vi "Auto Trans.vi"(0 "Scene Object In":refnum<vi>, 1 "Psi":dbl(slide) step=1.0 scale=-110.0..110.0, 2 "Psi i":dbl(slide) step=1.0 scale=-110.0..110.0, 3 "Boolean":bool, 5 "Base":refnum<vi>, 7 "Gimbal":refnum<vi>, 9 "Telescope":refnum<vi>, 11 "error in (no error)":errorcluster, 12 "Theta":dbl(slide) step=1.0 scale=-110.0..110.0, 13 "Theta i":dbl(slide) step=1.0 scale=-110.0..110.0) -> (4 "Scene Object Out":refnum<vi>, 15 "error out":errorcluster)   [LabVIEW 2015]
uses:
  <vilib>/picture/3D Picture Control/NI_3D Picture Control.lvlib
panel:
  out "Delta Psi 2":dbl
  out "Delta Psi":dbl
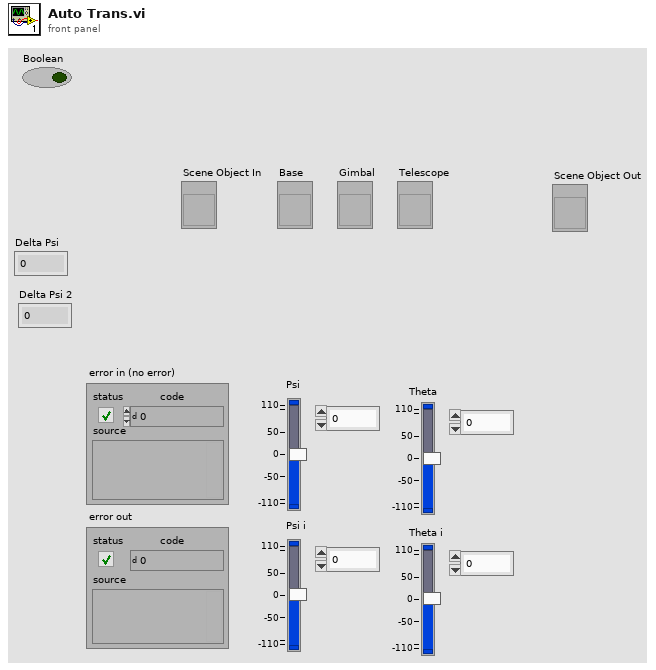
[diagram p1: front panel]
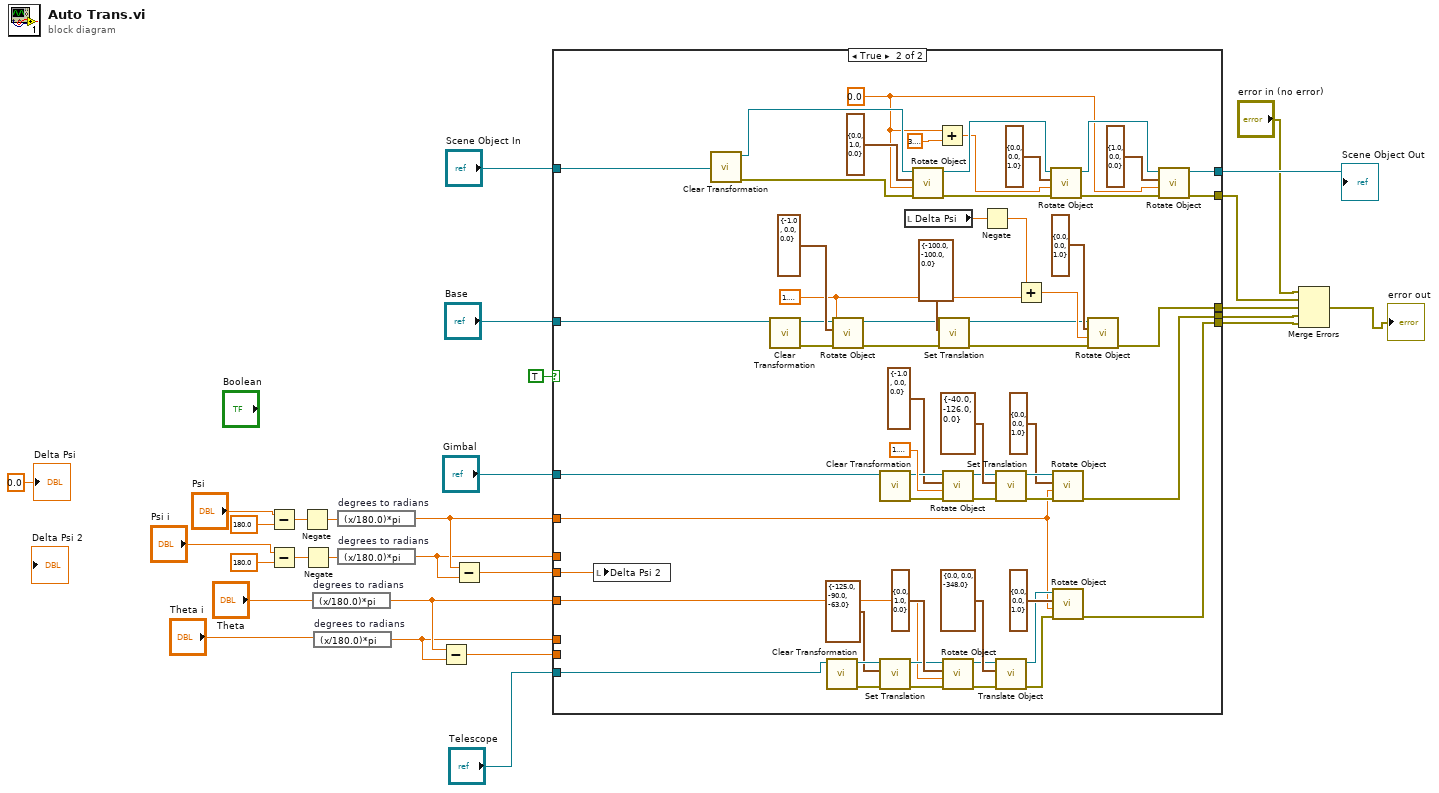
[diagram p0: block diagram]
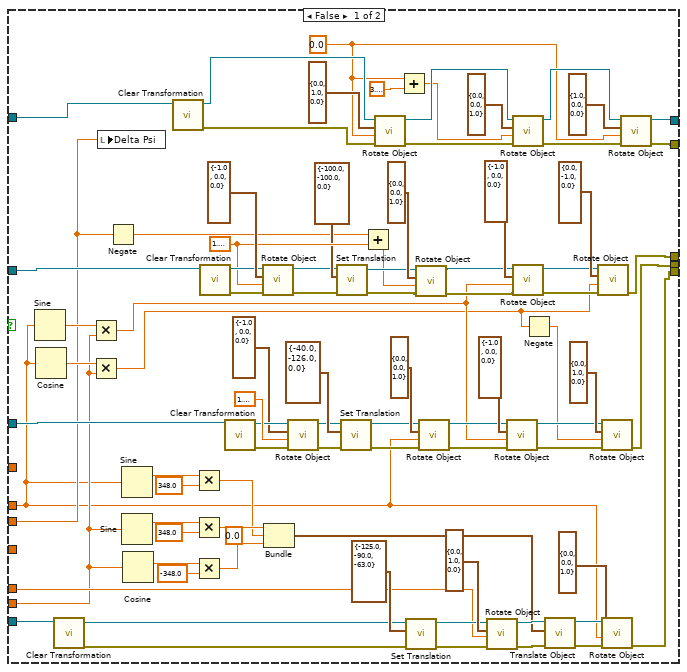
[diagram p2: hidden frame]
diagram:
  n1 = Subtract(x="Psi", y=180.0) -> (x-y=w5:dbl)
  n2 = Subtract(x="Psi i", y=180.0) -> (x-y=w3:dbl)
  n3 = Negate(x=w5) -> (-x=w6:dbl)
  n4 = Negate(x=w3) -> (-x=w4:dbl)
  n5 = expression code="(x/180.0)*pi" "degrees to radians"("Theta") -> (w12:dbl)
  n6 = expression code="(x/180.0)*pi" "degrees to radians"("Theta i") -> (w11:dbl)
  n7 = expression code="(x/180.0)*pi" "degrees to radians"(w6) -> (w10:dbl)
  n8 = expression code="(x/180.0)*pi" "degrees to radians"(w4) -> (w9:dbl)
  n9 = Subtract(x=w12, y=w11) -> (x-y=w7:dbl)
  n10 = Subtract(x=w10, y=w9) -> (x-y=w8:dbl)
  n11 = case shown="True" TRUE {
    tunnel: [w79 w161] -> w29
    tunnel: [w78 w160] -> w28
    tunnel: "Scene Object In" -> [w80 w159]
    tunnel: [w69 w120] -> w24
    tunnel: [w77 w132] -> w23
    tunnel: [w76 w131] -> w22
    tunnel: "Base" -> [w75 w130]
    tunnel: "Gimbal" -> [w74 w129]
    tunnel: "Telescope" -> [w73 w128]
    tunnel: w12 -> [_ w127]
    tunnel: w10 -> [_ w126]
    tunnel: w9 -> [w30 _]
    tunnel: w11 -> [w71 _]
    tunnel: w8 -> [w32 w123]
    tunnel: w7 -> [w43 _]
    frame False {
      (unwired) 0.0 ("y")
      w70 = 1.5707963267948966
      w103 = 0.0 ("x")
      n12 = Sine(x=w30) -> (sin(x)=w48:dbl)
      n13 = Cosine(x=w30) -> (cos(x)=w49:dbl)
      n14 = call <vilib>:"Clear Transformation.vi"("Object Refnum In"=w73) -> ("error out"=w88:errorcluster, "Object Refnum Out"=w72:refnum<vi>)  [unwired: 1 in, 8 out]
      n15 = Multiply(x=w48, y=w43) -> (x*y=w46:dbl)
      n16 = Multiply(x=w49, y=w43) -> (x*y=w44:dbl)
      n17 = local write "Delta Psi"(w32) -> ()
      n18 = Negate(x=w32) -> (-x=w35:dbl)
      n19 = Sine(x=w30) -> (sin(x)=w33:dbl)
      n20 = Sine(x=w43) -> (sin(x)=w41:dbl)
      n21 = Cosine(x=w43) -> (cos(x)=w39:dbl)
      n22 = call <vilib>:"Clear Transformation.vi"("Object Refnum In"=w80) -> ("error out"=w112:errorcluster, "Object Refnum Out"=w113:refnum<vi>)  [unwired: 1 in, 8 out]
      n23 = Multiply(x=w33, y=348.0) -> (x*y=w31:dbl)
      n24 = Multiply(x=w41, y=348.0) -> (x*y=w38:dbl)
      n25 = Multiply(x=w39, y=-348.0) -> (x*y=w37:dbl)
      n26 = call <vilib>:"Clear Transformation.vi"("Object Refnum In"=w75) -> ("error out"=w97:errorcluster, "Object Refnum Out"=w98:refnum<vi>)  [unwired: 1 in, 8 out]
      n27 = call <vilib>:"Clear Transformation.vi"("Object Refnum In"=w74) -> ("error out"=w94:errorcluster, "Object Refnum Out"=w95:refnum<vi>)  [unwired: 1 in, 8 out]
      n28 = call <vilib>:"Rotate Object.vi"("error in (no error)"=w97, "Angle"=w70, "Axis"=cluster{"X":sgl, "Y":sgl, "Z":sgl} {"X"=-1.0, "Y"=0.0, "Z"=0.0}, "Scene.Object In"=w98) -> ("error out"=w66:errorcluster, "Scene.Object Out"=w67:refnum<vi>)  [unwired: 6 in]
      n29 = Bundle(w38, w31, w37) -> (w36:cluster{dbl, dbl, dbl})  [unwired: 1 in]
      n30 = call <vilib>:"Rotate Object.vi"("error in (no error)"=w94, "Angle"=1.5707963267948966, "Axis"=cluster{"X":sgl, "Y":sgl, "Z":sgl} {"X"=-1.0, "Y"=0.0, "Z"=0.0}, "Scene.Object In"=w95) -> ("error out"=w92:errorcluster, "Scene.Object Out"=w93:refnum<vi>)  [unwired: 6 in]
      n31 = call <vilib>:"Set Translation.vi"("error in (no error)"=w66, "Translation"=cluster{"X":sgl, "Y":sgl, "Z":sgl} {"X"=-100.0, "Y"=-100.0, "Z"=0.0}, "Scene Object"=w67) -> ("error out"=w53:errorcluster, "Translated Object"=w50:refnum<vi>)  [unwired: 7 in]
      n32 = call <vilib>:"Set Translation.vi"("error in (no error)"=w92, "Translation"=cluster{"X":sgl, "Y":sgl, "Z":sgl} {"X"=-40.0, "Y"=-126.0, "Z"=0.0} ("Translation G"), "Scene Object"=w93) -> ("error out"=w58:errorcluster, "Translated Object"=w55:refnum<vi>)  [unwired: 7 in]
      n33 = Add(x=w35, y=w70) -> (x+y=w47:dbl)
      n34 = call <vilib>:"Rotate Object.vi"("error in (no error)"=w112, "Angle"=w103, "Axis"=cluster{"X":sgl, "Y":sgl, "Z":sgl} {"X"=0.0, "Y"=1.0, "Z"=0.0}, "Scene.Object In"=w113) -> ("error out"=w109:errorcluster, "Scene.Object Out"=w110:refnum<vi>)  [unwired: 6 in]
      n35 = Add(x=w103, y=3.141592653589793) -> (x+y=w104:dbl)
      n36 = call <vilib>:"Set Translation.vi"("error in (no error)"=w88, "Translation"=cluster{"X":sgl, "Y":sgl, "Z":sgl} {"X"=-125.0, "Y"=-90.0, "Z"=-63.0} ("Translation T1"), "Scene Object"=w72) -> ("error out"=w86:errorcluster, "Translated Object"=w87:refnum<vi>)  [unwired: 7 in]
      n37 = call <vilib>:"Rotate Object.vi"("error in (no error)"=w53, "Angle"=w47, "Axis"=cluster{"X":sgl, "Y":sgl, "Z":sgl} {"X"=0.0, "Y"=0.0, "Z"=1.0}, "Scene.Object In"=w50) -> ("error out"=w52:errorcluster, "Scene.Object Out"=w51:refnum<vi>)  [unwired: 6 in]
      n38 = call <vilib>:"Rotate Object.vi"("error in (no error)"=w58, "Angle"=w30, "Axis"=cluster{"X":sgl, "Y":sgl, "Z":sgl} {"X"=0.0, "Y"=0.0, "Z"=1.0}, "Scene.Object In"=w55) -> ("error out"=w57:errorcluster, "Scene.Object Out"=w56:refnum<vi>)  [unwired: 6 in]
      n39 = call <vilib>:"Rotate Object.vi"("error in (no error)"=w86, "Angle"=w71, "Axis"=cluster{"X":sgl, "Y":sgl, "Z":sgl} {"X"=0.0, "Y"=1.0, "Z"=0.0}, "Scene.Object In"=w87) -> ("error out"=w89:errorcluster, "Scene.Object Out"=w90:refnum<vi>)  [unwired: 6 in]
      n40 = call <vilib>:"Rotate Object.vi"("error in (no error)"=w57, "Angle"=w46, "Axis"=cluster{"X":sgl, "Y":sgl, "Z":sgl} {"X"=-1.0, "Y"=0.0, "Z"=0.0}, "Scene.Object In"=w56) -> ("error out"=w65:errorcluster, "Scene.Object Out"=w64:refnum<vi>)  [unwired: 6 in]
      n41 = call <vilib>:"Rotate Object.vi"("error in (no error)"=w109, "Angle"=w104, "Axis"=cluster{"X":sgl, "Y":sgl, "Z":sgl} {"X"=0.0, "Y"=0.0, "Z"=1.0}, "Scene.Object In"=w110) -> ("error out"=w107:errorcluster, "Scene.Object Out"=w106:refnum<vi>)  [unwired: 6 in]
      n42 = call <vilib>:"Rotate Object.vi"("error in (no error)"=w52, "Angle"=w46, "Axis"=cluster{"X":sgl, "Y":sgl, "Z":sgl} {"X"=-1.0, "Y"=0.0, "Z"=0.0}, "Scene.Object In"=w51) -> ("error out"=w60:errorcluster, "Scene.Object Out"=w61:refnum<vi>)  [unwired: 6 in]
      n43 = Negate(x=w44) -> (-x=w45:dbl)
      n44 = call <vilib>:"Translate Object.vi"("error in (no error)"=w89, "Translation"=w36, "Scene.Object In"=w90) -> ("error out"=w82:errorcluster, "Scene.Object Out"=w83:refnum<vi>)  [unwired: 7 in]
      n45 = call <vilib>:"Rotate Object.vi"("error in (no error)"=w60, "Angle"=w44, "Axis"=cluster{"X":sgl, "Y":sgl, "Z":sgl} {"X"=0.0, "Y"=-1.0, "Z"=0.0}, "Scene.Object In"=w61) -> ("error out"=w69:errorcluster)  [unwired: 6 in, 1 out]
      n46 = call <vilib>:"Rotate Object.vi"("error in (no error)"=w65, "Angle"=w45, "Axis"=cluster{"X":sgl, "Y":sgl, "Z":sgl} {"X"=0.0, "Y"=1.0, "Z"=0.0}, "Scene.Object In"=w64) -> ("error out"=w77:errorcluster)  [unwired: 6 in, 1 out]
      n47 = call <vilib>:"Rotate Object.vi"("error in (no error)"=w82, "Angle"=w30, "Axis"=cluster{"X":sgl, "Y":sgl, "Z":sgl} {"X"=0.0, "Y"=0.0, "Z"=1.0}, "Scene.Object In"=w83) -> ("error out"=w76:errorcluster)  [unwired: 6 in, 1 out]
      n48 = call <vilib>:"Rotate Object.vi"("error in (no error)"=w107, "Angle"=w103, "Axis"=cluster{"X":sgl, "Y":sgl, "Z":sgl} {"X"=1.0, "Y"=0.0, "Z"=0.0}, "Scene.Object In"=w106) -> ("error out"=w78:errorcluster, "Scene.Object Out"=w79:refnum<vi>)  [unwired: 6 in]
    }
    frame True {
      w124 = 1.5707963267948966
      w162 = 0.0 ("x")
      n49 = local write "Delta Psi 2"(w123) -> ()
      n50 = call <vilib>:"Clear Transformation.vi"("Object Refnum In"=w159) -> ("error out"=w171:errorcluster, "Object Refnum Out"=w172:refnum<vi>)  [unwired: 1 in, 8 out]
      n51 = call <vilib>:"Clear Transformation.vi"("Object Refnum In"=w130) -> ("error out"=w151:errorcluster, "Object Refnum Out"=w152:refnum<vi>)  [unwired: 1 in, 8 out]
      n52 = call <vilib>:"Clear Transformation.vi"("Object Refnum In"=w128) -> ("error out"=w140:errorcluster, "Object Refnum Out"=w141:refnum<vi>)  [unwired: 1 in, 8 out]
      n53 = call <vilib>:"Rotate Object.vi"("error in (no error)"=w151, "Angle"=w124, "Axis"=cluster{"X":sgl, "Y":sgl, "Z":sgl} {"X"=-1.0, "Y"=0.0, "Z"=0.0}, "Scene.Object In"=w152) -> ("error out"=w117:errorcluster, "Scene.Object Out"=w118:refnum<vi>)  [unwired: 6 in]
      n54 = call <vilib>:"Clear Transformation.vi"("Object Refnum In"=w129) -> ("error out"=w148:errorcluster, "Object Refnum Out"=w149:refnum<vi>)  [unwired: 1 in, 8 out]
      n55 = call <vilib>:"Set Translation.vi"("error in (no error)"=w140, "Translation"=cluster{"X":sgl, "Y":sgl, "Z":sgl} {"X"=-125.0, "Y"=-90.0, "Z"=-63.0} ("Translation T1"), "Scene Object"=w141) -> ("error out"=w138:errorcluster, "Translated Object"=w139:refnum<vi>)  [unwired: 7 in]
      n56 = local read "Delta Psi"() -> (w122:dbl)
      n57 = call <vilib>:"Rotate Object.vi"("error in (no error)"=w171, "Angle"=w162, "Axis"=cluster{"X":sgl, "Y":sgl, "Z":sgl} {"X"=0.0, "Y"=1.0, "Z"=0.0}, "Scene.Object In"=w172) -> ("error out"=w168:errorcluster, "Scene.Object Out"=w169:refnum<vi>)  [unwired: 6 in]
      n58 = Add(x=w162, y=3.141592653589793) -> (x+y=w163:dbl)
      n59 = call <vilib>:"Set Translation.vi"("error in (no error)"=w117, "Translation"=cluster{"X":sgl, "Y":sgl, "Z":sgl} {"X"=-100.0, "Y"=-100.0, "Z"=0.0}, "Scene Object"=w118) -> ("error out"=w115:errorcluster, "Translated Object"=w116:refnum<vi>)  [unwired: 7 in]
      n60 = call <vilib>:"Rotate Object.vi"("error in (no error)"=w148, "Angle"=1.5707963267948966, "Axis"=cluster{"X":sgl, "Y":sgl, "Z":sgl} {"X"=-1.0, "Y"=0.0, "Z"=0.0}, "Scene.Object In"=w149) -> ("error out"=w146:errorcluster, "Scene.Object Out"=w147:refnum<vi>)  [unwired: 6 in]
      n61 = call <vilib>:"Rotate Object.vi"("error in (no error)"=w138, "Angle"=w127, "Axis"=cluster{"X":sgl, "Y":sgl, "Z":sgl} {"X"=0.0, "Y"=1.0, "Z"=0.0}, "Scene.Object In"=w139) -> ("error out"=w142:errorcluster, "Scene.Object Out"=w143:refnum<vi>)  [unwired: 6 in]
      n62 = Negate(x=w122) -> (-x=w121:dbl)
      n63 = call <vilib>:"Set Translation.vi"("error in (no error)"=w146, "Translation"=cluster{"X":sgl, "Y":sgl, "Z":sgl} {"X"=-40.0, "Y"=-126.0, "Z"=0.0} ("Translation G"), "Scene Object"=w147) -> ("error out"=w156:errorcluster, "Translated Object"=w157:refnum<vi>)  [unwired: 7 in]
      n64 = call <vilib>:"Translate Object.vi"("error in (no error)"=w142, "Translation"=cluster{"X":sgl, "Y":sgl, "Z":sgl} {"X"=0.0, "Y"=0.0, "Z"=-348.0} ("Translation T2"), "Scene.Object In"=w143) -> ("error out"=w134:errorcluster, "Scene.Object Out"=w135:refnum<vi>)  [unwired: 7 in]
      n65 = Add(x=w121, y=w124) -> (x+y=w125:dbl)
      n66 = call <vilib>:"Rotate Object.vi"("error in (no error)"=w168, "Angle"=w163, "Axis"=cluster{"X":sgl, "Y":sgl, "Z":sgl} {"X"=0.0, "Y"=0.0, "Z"=1.0}, "Scene.Object In"=w169) -> ("error out"=w166:errorcluster, "Scene.Object Out"=w165:refnum<vi>)  [unwired: 6 in]
      n67 = call <vilib>:"Rotate Object.vi"("error in (no error)"=w156, "Angle"=w126, "Axis"=cluster{"X":sgl, "Y":sgl, "Z":sgl} {"X"=0.0, "Y"=0.0, "Z"=1.0}, "Scene.Object In"=w157) -> ("error out"=w132:errorcluster)  [unwired: 6 in, 1 out]
      n68 = call <vilib>:"Rotate Object.vi"("error in (no error)"=w134, "Angle"=w126, "Axis"=cluster{"X":sgl, "Y":sgl, "Z":sgl} {"X"=0.0, "Y"=0.0, "Z"=1.0}, "Scene.Object In"=w135) -> ("error out"=w131:errorcluster)  [unwired: 6 in, 1 out]
      n69 = call <vilib>:"Rotate Object.vi"("error in (no error)"=w115, "Angle"=w125, "Axis"=cluster{"X":sgl, "Y":sgl, "Z":sgl} {"X"=0.0, "Y"=0.0, "Z"=1.0}, "Scene.Object In"=w116) -> ("error out"=w120:errorcluster)  [unwired: 6 in, 1 out]
      n70 = call <vilib>:"Rotate Object.vi"("error in (no error)"=w166, "Angle"=w162, "Axis"=cluster{"X":sgl, "Y":sgl, "Z":sgl} {"X"=1.0, "Y"=0.0, "Z"=0.0}, "Scene.Object In"=w165) -> ("error out"=w160:errorcluster, "Scene.Object Out"=w161:refnum<vi>)  [unwired: 6 in]
    }
  }
  "Scene Object Out" <- w29
  n71 = Merge Errors("error in (no error)", w28, w24, w23, w22) -> (→"error out":errorcluster)
  "Delta Psi" <- 0.0 ("Delta Psi")
